vi "Util.Cmprs.LZW.CU.StringsTable.vi"(6 "Bits":i32, 8 "error in (no error)":errorcluster, 9 "Codes in":i16[](array[numeric]), 10 "Chars in":u8[](array[numeric]), 11 "Pack":bool) -> (0 "error out":errorcluster, 1 "Chars out":u8[](array[numeric]), 2 "Codes out":i16[](array[numeric]))   [LabVIEW 2014]
panel:
  out "Unpacked":string[](array[string])
  out "Packed":string[](array[string])
  # "Util.Cmprs.LZW.CU.StringsTable.vi\n\nCompresses/Decompresses data-stream to/from LZW codes array.\n\nPlease visit http://www.OpenG.org to learn about the\nOpen Source LabVIEW software movement.\n\nNOTICE -- YOU MUST LEAVE THIS NOTICE IN PLACE.  PER THE TERMS OF THE LICENSE BELOW, YOU MAY SUBLICENSE THIS SOFTWARE \nIN ANY WAY THAT DOES NOT CONFLICT WITH THIS LICENSE.\n\n### BSD License (http://www.opensource.org/licenses/bsd-license.php) Begin ###\n \nCopyright (c) 2007, Bill Clench <bclench@yahoo.com>\n\nAll rights reserved.\n\nRedistribution and use in source and binary forms, with or without modification, are permitted provided that the following conditions are met:\n\n    * Redistributions of source code must retain the above copyright notice, this list of conditions and the following disclaimer.\n    * Redistributions in binary form must reproduce the above copyright notice, this list of conditions and the following disclaimer in the \n       documentation and/or other materials provided with the distribution.\n\nTHIS SOFTWARE IS PROVIDED BY THE COPYRIGHT HOLDERS AND CONTRIBUTORS \"AS IS\" AND ANY EXPRESS OR IMPLIED WARRANTIES, \nINCLUDING, BUT NOT LIMITED TO, THE IMPLIED WARRANTIES OF MERCHANTABILITY AND FITNESS FOR A PARTICULAR PURPOSE ARE \nDISCLAIMED. IN NO EVENT SHALL THE COPYRIGHT OWNER OR CONTRIBUTORS BE LIABLE FOR ANY DIRECT, INDIRECT, INCIDENTAL,\n SPECIAL, EXEMPLARY, OR CONSEQUENTIAL DAMAGES (INCLUDING, BUT NOT LIMITED TO, PROCUREMENT OF SUBSTITUTE GOODS OR \nSERVICES; LOSS OF USE, DATA, OR PROFITS; OR BUSINESS INTERRUPTION) HOWEVER CAUSED AND ON ANY THEORY OF LIABILITY, \nWHETHER IN CONTRACT, STRICT LIABILITY, OR TORT (INCLUDING NEGLIGENCE OR OTHERWISE) ARISING IN ANY WAY OUT OF THE USE \nOF THIS SOFTWARE, EVEN IF ADVISED OF THE POSSIBILITY OF SUCH DAMAGE.\n\n### BSD License End ###"
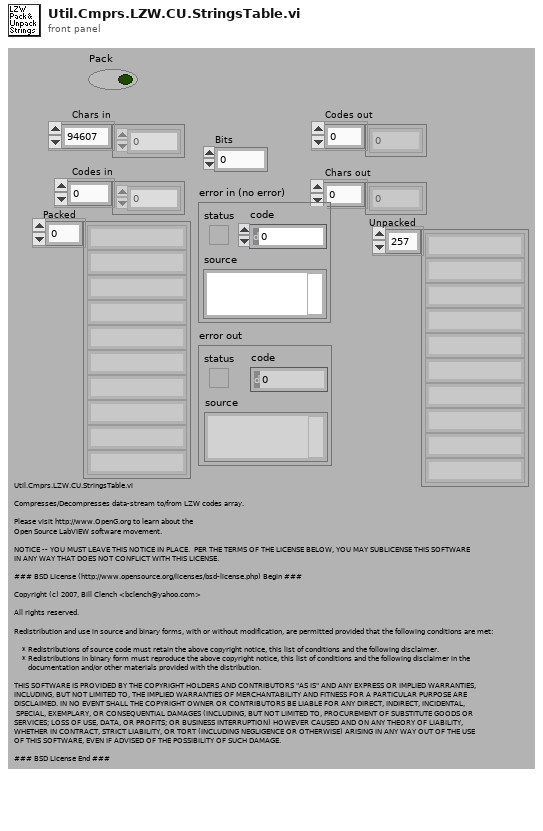
[diagram p1: front panel]
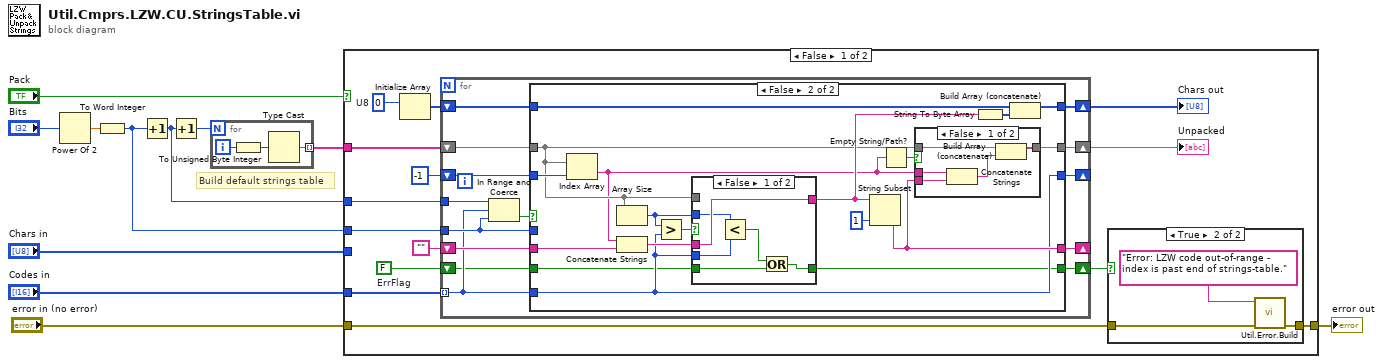
[diagram p0: block diagram]
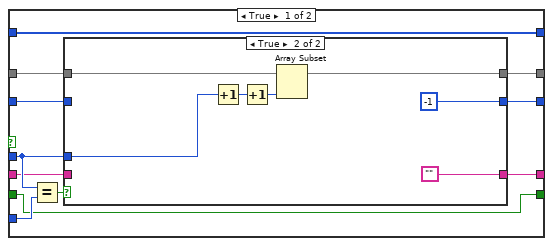
[diagram p3: hidden frame]
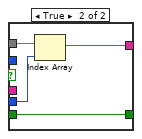
[diagram p6: hidden frame]
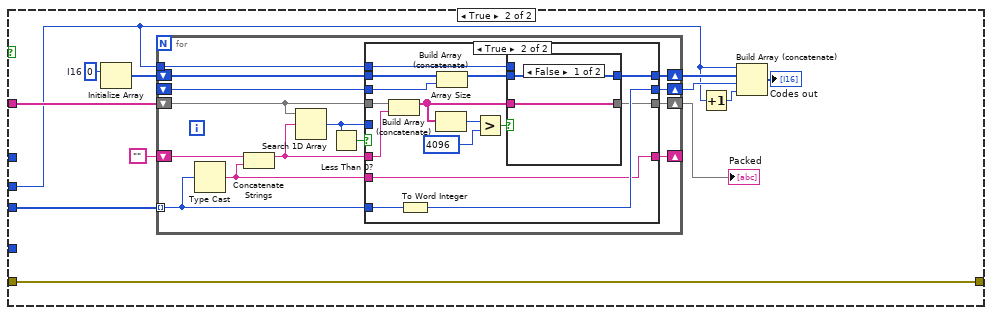
[diagram p7: hidden frame]
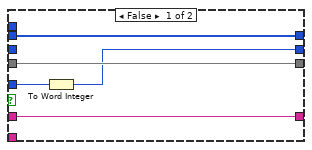
[diagram p8: hidden frame]
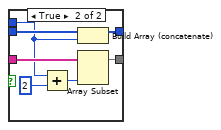
[diagram p9: hidden frame]
diagram:
  # "Build default strings table"
  n1 = Power Of 2(x="Bits") -> (2^x=w7:dbl)
  n2 = To Word Integer(number=w7) -> (16bit integer=w4:i16)
  n3 = Increment(x=w4) -> (x+1=w3:i16)
  n4 = Increment(x=w3) -> (x+1=w5:i16)
  n5 = for {
    N: w5 -> [_]
    tunnel: [w14] -> w6 mode=indexing
    i -> [w12]
    n6 = To Unsigned Byte Integer(number=w12) -> (unsigned 8bit integer=w13:u8)
    n7 = Type Cast(x=w13) -> (*(type *) &x=w14:string)  [unwired: 1 in]
  }
  n8 = case shown="False" "Pack" {
    tunnel: "Chars in" -> [_ w113]
    tunnel: w6 -> [w28 w111]
    tunnel: "Codes in" -> [w24 _]
    tunnel: w4 -> [w19 w103]
    tunnel: w3 -> [w20 _]
    tunnel: [w15 w102] -> w2
    tunnel: "error in (no error)" -> [w16 w102]
    frame False {
      w18 = FALSE  # ErrFlag
      w26 = u8 0  # U8
      n9 = Initialize Array(w26) -> (w27:u8[])  [unwired: 1 in]
      n10 = for {
        shift-right: [w43] -> w23
        shift-left: w28 -> [w44]
        shift-right: [w39] -> _
        shift-left: "" -> [w40]
        tunnel: w24 -> [w35] mode=indexing
        shift-right: [w42] -> w21
        shift-left: w27 -> [w46]
        shift-right: [w41] -> _
        shift-left: i16 -1 -> [w45]
        tunnel: w20 -> [w38]
        tunnel: w19 -> [w37]
        shift-right: [w33] -> w17
        shift-left: w18 -> [w34]
        n11 = In Range and Coerce(upper limit=w38, x=w35, lower limit=w37) -> (In Range?=w36:bool)  [unwired: 1 out]
        n12 = case shown="False" w36 {
          tunnel: w46 -> [w57 w83]
          tunnel: w45 -> [w49 w77]
          tunnel: w44 -> [w56 w73]
          tunnel: [w55 w82] -> w43
          tunnel: [w57 w81] -> w42
          tunnel: [w53 w71] -> w41
          tunnel: w40 -> [w48 w76]
          tunnel: [w54 w74] -> w39
          tunnel: w35 -> [w51 w71]
          tunnel: w37 -> [w52 _]
          tunnel: w34 -> [w47 w69]
          tunnel: [w47 w68] -> w33
          frame True {
            n13 = Equal?(x=w52, y=w51) -> (x = y?=w50:bool)
            n14 = case shown="True" w50 {
              tunnel: w56 -> [w60 w67]
              tunnel: [w60 w66] -> w55
              tunnel: [w58 ""] -> w54
              tunnel: [w59 i16 -1] -> w53
              tunnel: w52 -> [_ w61]
              tunnel: w49 -> [w59 _]
              tunnel: w48 -> [w58 _]
              frame False {
              }
              frame True {
                n15 = Increment(x=w61) -> (x+1=w63:i16)
                n16 = Increment(x=w63) -> (x+1=w62:i16)
                n17 = Array Subset(array=w67, length=w62) -> (w66:string[])  [unwired: 1 in]
              }
            }
          }
          frame False {
            n18 = Index Array(array=w73, index=w77) -> (element=w72:string)
            n19 = Array Size(array=w73) -> (size(s)=w70:i32)
            n20 = Concatenate Strings(w72, w76) -> (w75:string)
            n21 = Greater?(x=w70, y=w71) -> (0:w85:bool)
            n22 = case shown="False" w85 {
              tunnel: w75 -> [w97 _]
              tunnel: [w97 w100] -> w78
              tunnel: w73 -> [_ w101]
              tunnel: w71 -> [w95 w99]
              tunnel: w70 -> [w96 _]
              tunnel: w69 -> [w94 w98]
              tunnel: [w92 w98] -> w68
              frame False {
                n23 = Less?(x=w96, y=w95) -> (x < y?=w93:bool)
                n24 = Or(x=w93, y=w94) -> (x .or. y?=w92:bool)
              }
              frame True {
                n25 = Index Array(array=w101, index=w99) -> (element=w100:string)
              }
            }
            n26 = String Subset(string=w78, length (rest)=1) -> (substring=w74:string)  [unwired: 1 in]
            n27 = Empty String/Path?(string/path=w72) -> (empty?=w80:bool)
            n28 = case shown="False" w80 {
              tunnel: w73 -> [w90 w91]
              tunnel: [w89 w91] -> w82
              tunnel: w74 -> [w86 _]
              tunnel: w72 -> [w88 _]
              frame False {
                n29 = Concatenate Strings(w88, w86) -> (w87:string)
                n30 = Build Array (concatenate)(w90, w87) -> (w89:string[])
              }
              frame True {
              }
            }
            n31 = String To Byte Array(string=w78) -> (unsigned byte array=w84:u8[])
            n32 = Build Array (concatenate)(w83, w84) -> (w81:u8[])
          }
        }
      }
      "Chars out" <- w21
      "Unpacked" <- w23
      n33 = case shown="True" w17 {
        tunnel: w16 -> [w29 w31]
        tunnel: [w29 w32] -> w15
        frame False {
        }
        frame True {
          n34 = call "Util.Error.Build.vi"("error in (no error)"=w31, "Source"="Error: LZW code out-of-range - index is past end of strings-table.") -> ("error out"=w32:errorcluster)  [unwired: 9 in]
        }
      }
    }
    frame True {
      w109 = i16 0  # I16
      n35 = Initialize Array(w109) -> (w110:i16[])  [unwired: 1 in]
      n36 = for {
        tunnel: w113 -> [w117] mode=indexing
        shift-right: [w116] -> _
        shift-left: "" -> [w120]
        shift-right: [w118] -> w105
        shift-left: w111 -> [w127]
        shift-right: [w124] -> w107
        shift-left: _ -> [w121]
        shift-right: [w122] -> w108
        shift-left: w110 -> [w123]
        tunnel: w103 -> [w114]
        n37 = Type Cast(x=w117) -> (*(type *) &x=w115:string)  [unwired: 1 in]
        n38 = Concatenate Strings(w120, w115) -> (w119:string)
        n39 = Search 1D Array(1D array=w127, element=w119) -> (index of element=w125:i32)  [unwired: 1 in]
        n40 = Less Than 0?(x=w125) -> (x < 0?=w126:bool)
        n41 = case shown="True" w126 {
          tunnel: w127 -> [w130 w146]
          tunnel: w125 -> [w132 _]
          tunnel: [w129 w143] -> w124
          tunnel: w123 -> [w131 w147]
          tunnel: [w131 w137] -> w122
          tunnel: w121 -> [_ w141]
          tunnel: w119 -> [w128 w145]
          tunnel: [w130 w139] -> w118
          tunnel: w117 -> [_ w144]
          tunnel: [w128 w142] -> w116
          tunnel: w115 -> [_ w142]
          tunnel: w114 -> [_ w133]
          frame False {
            n42 = To Word Integer(number=w132) -> (16bit integer=w129:i16)
          }
          frame True {
            n43 = Build Array (concatenate)(w146, w145) -> (w140:string[])
            n44 = To Word Integer(number=w144) -> (16bit integer=w143:i16)
            n45 = Array Size(array=w140) -> (size(s)=w136:i32)
            n46 = Build Array (concatenate)(w147, w141) -> (w138:i16[])
            n47 = Greater?(x=w136, y=4096) -> (0:w134:bool)
            n48 = case shown="False" w134 {
              tunnel: w140 -> [w149 w156]
              tunnel: [w149 w155] -> w139
              tunnel: w138 -> [w148 w154]
              tunnel: [w148 w153] -> w137
              tunnel: w133 -> [_ w151]
              frame False {
              }
              frame True {
                n49 = Add(x=w151, y=i16 2) -> (x+y=w152:i16)
                n50 = Build Array (concatenate)(w154, w151) -> (w153:i16[])
                n51 = Array Subset(array=w156, length=w152) -> (w155:string[])  [unwired: 1 in]
              }
            }
          }
        }
      }
      "Packed" <- w105
      n52 = Increment(x=w103) -> (x+1=w104:i16)
      n53 = Build Array (concatenate)(w103, w108, w107, w104) -> (→"Codes out":i16[])
    }
  }
  "error out" <- w2
